vi "MccHat_Global.vi"() -> ()   [LabVIEW 2019]
panel:
  out "MccHat_ST":u32(colorbox)
  out "MccHat_P":dbl format="%.1f"
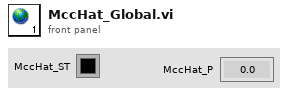
[diagram p1: front panel]
diagram:
